vi "Orbit WIthout PID.vi"() -> ()   [LabVIEW 2025]
uses:
  <vilib>/Rock Robotics/Network Tables/NT Read Float Array.vi
  swerve-template/Type Definitions/Data/Robot Velocities.ctl
panel:
  in  "test values":sgl[](array[numeric])
  out "Output Velocities":T1
  in  "Input Velocities":T1
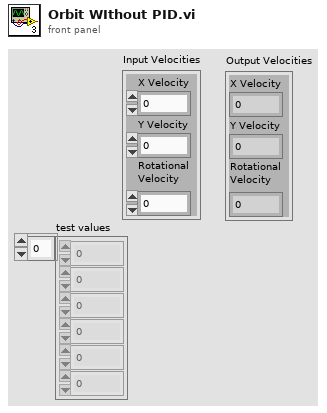
[diagram p1: front panel]
types:
  T1 = typedef "Robot Velocities.ctl" = cluster{"X Velocity":dbl, "Y Velocity":dbl, "Rotational \nVelocity":dbl}
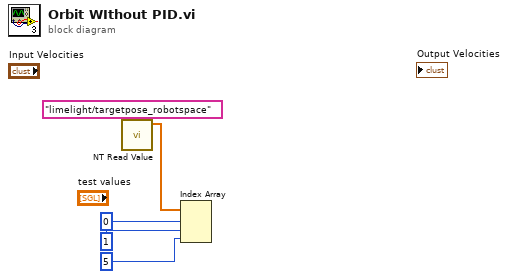
[diagram p0: block diagram]
diagram:
  n1 = call-poly <vilib>:"NT Read Value.vi"("name"="limelight/targetpose_robotspace") -> ("value"=w1:sgl[])  [unwired: 8 in, 2 out]
  n2 = Index Array(array=w1, index #1=0 ("index"), index #2=1 ("index"), index #3=5 ("index")) -> ()  [unwired: 3 out]
